vi "cal data.vi"(9 "输入簇":T1, 10 "range":enum16{"±1V", "±5V"}(ring), 11 "data":dbl[](array[numeric])) -> (2 "data out":dbl[](array[numeric]))   [LabVIEW 2011]
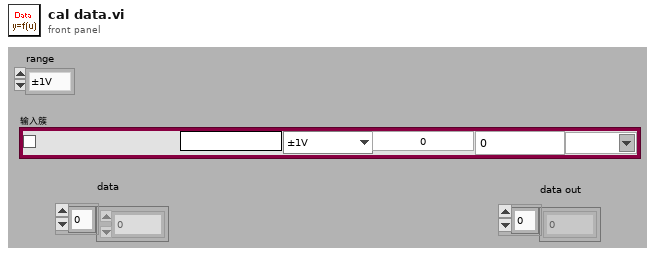
[diagram p1: front panel]
types:
  T1 = typedef "Acceleration Channel Config_Ctrls-某型振动实验台测试系统.ctl" = cluster{"Enable":bool, "Name":string, "range":enum16{"±1V", "±5V"}, "SensValue":dbl, "PhysicalName":string, "off":dbl, "Sensunits":string}
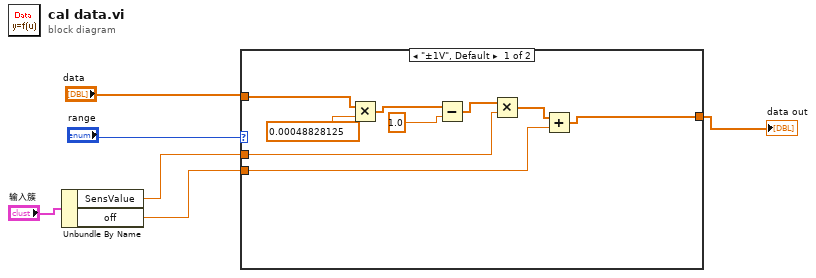
[diagram p0: block diagram]
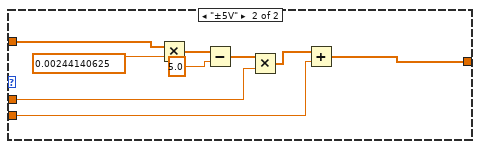
[diagram p2: hidden frame]
diagram:
  n1 = Unbundle By Name("输入簇") -> ("SensValue"=w3:dbl, "off"=w2:dbl)
  n2 = case shown="\"±1V\", Default" "range" {
    tunnel: w3 -> [w9 w18]
    tunnel: w2 -> [w14 w16]
    tunnel: "data" -> [w13 w24]
    tunnel: [w7 w22] -> w6
    frame "±1V", Default {
      n3 = Multiply(x=w13, y=0.00048828125) -> (x*y=w12:dbl[])
      n4 = Subtract(x=w12, y=1.0) -> (x-y=w10:dbl[])
      n5 = Multiply(x=w10, y=w9) -> (x*y=w8:dbl[])
      n6 = Add(x=w8, y=w14) -> (x+y=w7:dbl[])
    }
    frame "±5V" {
      n7 = Multiply(x=w24, y=0.00244140625) -> (x*y=w23:dbl[])
      n8 = Subtract(x=w23, y=5.0) -> (x-y=w19:dbl[])
      n9 = Multiply(x=w19, y=w18) -> (x*y=w17:dbl[])
      n10 = Add(x=w17, y=w16) -> (x+y=w22:dbl[])
    }
  }
  "data out" <- w6
